vi "rs3 get error message.vi"(8 "error in (no error)":errorcluster, 11 "error in":u64) -> (0 "error out":errorcluster, 2 "error out":u64, 3 "error message":string)   [LabVIEW 2019, in "libRealSense3.lvlib"]
doc: "const char * rs_get_error_message (const rs_error * error);"
uses:
  libRealSense3.lvlib
  realsense2.dll
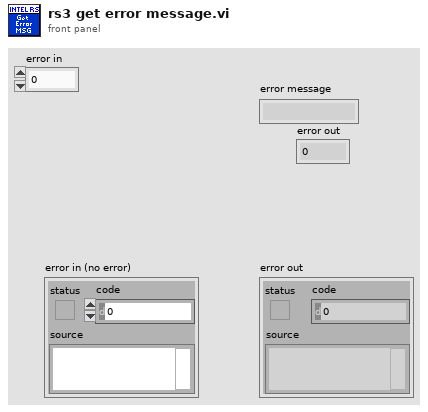
[diagram p1: front panel]
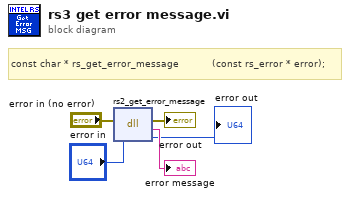
[diagram p0: block diagram]
diagram:
  # "const char * rs_get_error_message           (const rs_error * error);"
  n1 = dll-call lib="C:/Users/morte/Documents/gitmoro/treadmill/RealSense for Labview ver. 2.33/realsense2.dll" fn="rs2_get_error_message"(error in="error in (no error)", "error"="error in") -> (error out=→"error out":errorcluster, "return type"=→"error message":string, "error"=→"error out":u64)  [unwired: 2 in, 1 out]
